vi "Open FPGA Session.vi"(7 "run when loaded (T)":bool=TRUE, 8 "error in":errorcluster, 10 "bitfile path":path, 11 "device address":string) -> (0 "error out":errorcluster, 2 "session out":u64, 3 "bitfile reference out":refnum<k20>)   [LabVIEW 2018, in "Scalar IO Operations.lvlib"]
uses:
  Scalar IO Operations.lvlib
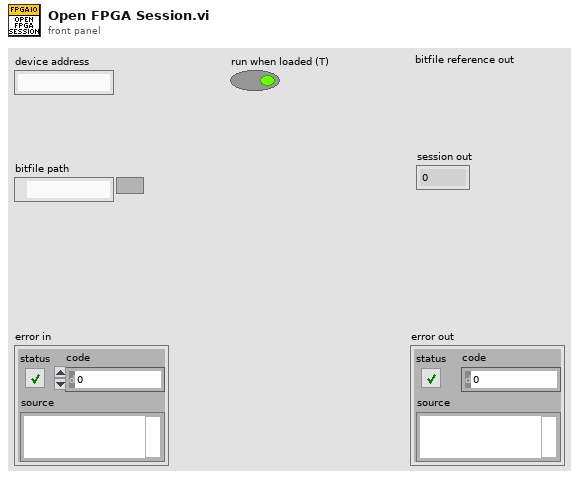
[diagram p1: front panel]
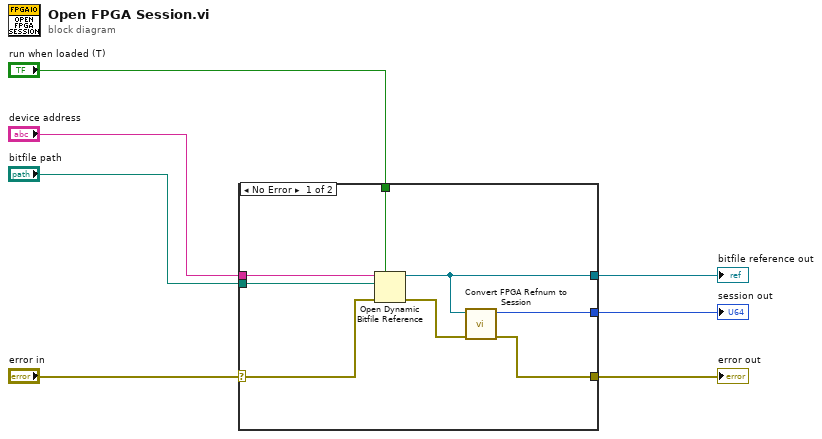
[diagram p0: block diagram]
diagram:
  n1 = case shown="No Error" "error in" {
    selector: "error in" -> [w11 w16]
    tunnel: "run when loaded (T)" -> [w15 _]
    tunnel: "device address" -> [w13 _]
    tunnel: "bitfile path" -> [w12 _]
    tunnel: [w10 w16] -> w2
    tunnel: [w9 _] -> w3
    tunnel: [w8 _] -> w1
    frame No Error {
      n2 = Open Dynamic Bitfile Reference(0:w13, 1:w12, 2:w15, 3:w11) -> (5:w8:refnum<k20>, 8:w14:errorcluster)  [unwired: 1 in]
      n3 = call "Convert FPGA Refnum to Session.vi"("error in (no error)"=w14, "fpga refnum in"=w8) -> ("error out"=w10:errorcluster, "session out"=w9:u64)  [unwired: 8 in]
    }
    frame Error {
    }
  }
  "session out" <- w3
  "error out" <- w2
  "bitfile reference out" <- w1
